vi "test - Arguments or Respsone.vi"(8 "error in (no error)":errorcluster, 11 "TestCase in":refnum<class "testcase-Supported-Datatype.lvclass">) -> (0 "error out":errorcluster, 3 "TestCase out":refnum<class "testcase-Supported-Datatype.lvclass">)   [LabVIEW 2017, in "testcase-Supported-Datatype.lvclass"]
uses:
  testcase-Supported-Datatype.lvclass
  3126c190-a873-4347-b4f7-a4a9805c9280.vi
  c9e66315-a3dc-45cf-9eb3-a329de137435.vi
  5e45644a-04d9-431d-85da-59447771591c.vi
  acccb231-0f0e-4c8a-8d12-71726bcd94d5.vi
  addons/API-String-Arugments-Support/_Support/Convert API String Arguments to Data(variant).vi
  <vilib>/addons/_JKI Toolkits/VI Tester/TestCase.llb/TestCase.lvclass
  C:/Program Files (x86)/National Instruments/LabVIEW 2017/vi.lib/addons/_JKI Toolkits/VI Tester/TestCase.llb/TestCase.lvclass
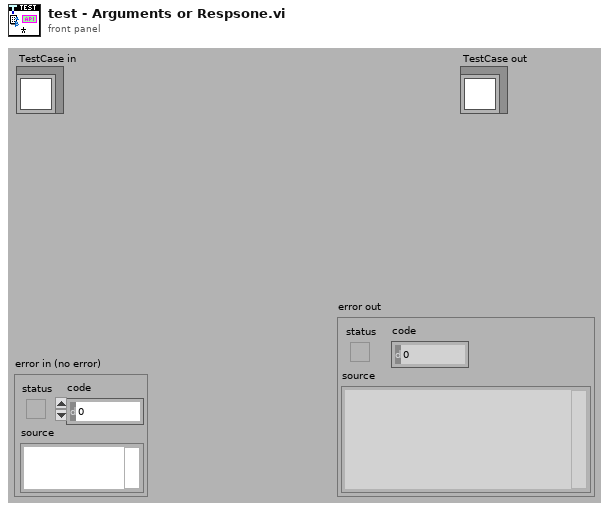
[diagram p1: front panel]
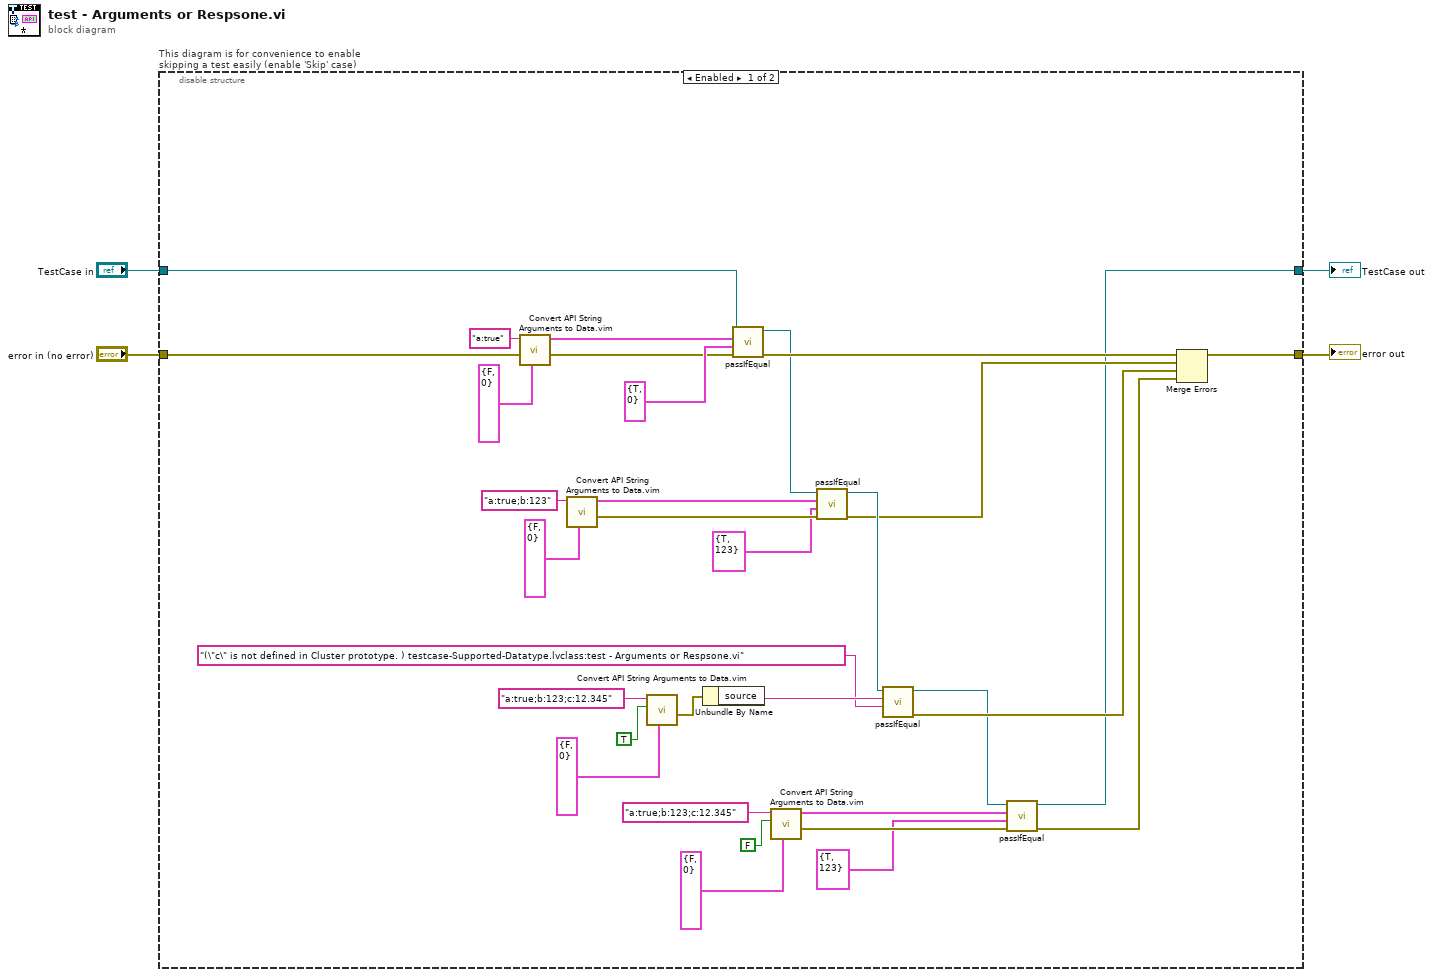
[diagram p0: block diagram]
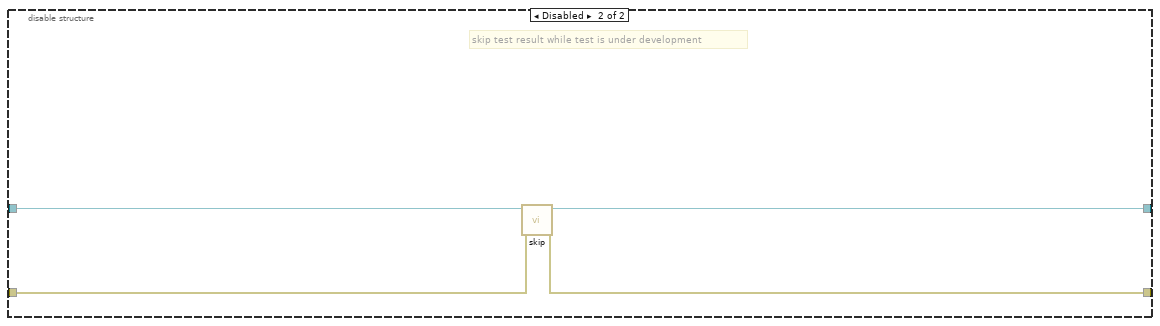
[diagram p2: hidden frame]
diagram:
  n1 = disable-structure "This diagram is for convenience to enable skipping a test easily (enable 'Skip' case)" shown="Enabled" {
    disable-tunnel: "TestCase in" -> [w37 w41]
    disable-tunnel: [w9 w39] -> w1
    disable-tunnel: [w36 w40] -> w3
    disable-tunnel: "error in (no error)" -> [w25 w38]
    frame Enabled {
      n2 = call "Convert API String Arguments to Data.vim"("Reference Type"=cluster{"a":bool, "b":i32} {"a"=FALSE, "b"=0}, "error in (no error)"=w25, "API String"="a:true" ("String")) -> ("error out"=w27:errorcluster, "Data"=w29:cluster{"a":bool, "b":i32})  [unwired: 5 in]
      n3 = call "Convert API String Arguments to Data.vim"("Reference Type"=cluster{"a":bool, "b":i32} {"a"=FALSE, "b"=0}, "API String"="a:true;b:123" ("String")) -> ("error out"=w22:errorcluster, "Data"=w20:cluster{"a":bool, "b":i32})  [unwired: 6 in]
      n4 = call "Convert API String Arguments to Data.vim"("Reference Type"=cluster{"a":bool, "b":i32} {"a"=FALSE, "b"=0}, "Strict Label Check? (T)"=TRUE ("Strict Label Check?(T)"), "API String"="a:true;b:123;c:12.345" ("String")) -> ("error out"=w7:errorcluster)  [unwired: 5 in, 1 out]
      n5 = Unbundle By Name(w7) -> ("source"=w6:string)
      n6 = call-dynamic "passIfEqual.vi"("error in (no error)"=w27, "y"=cluster{"a":bool, "b":i32} {"a"=TRUE, "b"=0} ("Data"), "x"=w29, "TestCase in"=w37) -> ("error out"=w26:errorcluster, "TestCase out"=w24:refnum<class "testcase-Supported-Datatype.lvclass">)  [unwired: 6 in]
      n7 = call "Convert API String Arguments to Data.vim"("Reference Type"=cluster{"a":bool, "b":i32} {"a"=FALSE, "b"=0}, "Strict Label Check? (T)"=FALSE ("Strict Label Check?(T)"), "API String"="a:true;b:123;c:12.345" ("String")) -> ("error out"=w15:errorcluster, "Data"=w13:cluster{"a":bool, "b":i32})  [unwired: 5 in]
      n8 = call-dynamic "passIfEqual.vi"("error in (no error)"=w22, "y"=cluster{"a":bool, "b":i32} {"a"=TRUE, "b"=123} ("Data 2"), "x"=w20, "TestCase in"=w24) -> ("error out"=w18:errorcluster, "TestCase out"=w23:refnum<class "testcase-Supported-Datatype.lvclass">)  [unwired: 6 in]
      n9 = call-dynamic "passIfEqual.vi"("y"="(\"c\" is not defined in Cluster prototype. ) testcase-Supported-Datatype.lvclass:test - Arguments or Respsone.vi" ("source"), "x"=w6, "TestCase in"=w23) -> ("error out"=w19:errorcluster, "TestCase out"=w10:refnum<class "testcase-Supported-Datatype.lvclass">)  [unwired: 7 in]
      n10 = call-dynamic "passIfEqual.vi"("error in (no error)"=w15, "y"=cluster{"a":bool, "b":i32} {"a"=TRUE, "b"=123} ("Data 3"), "x"=w13, "TestCase in"=w10) -> ("error out"=w8:errorcluster, "TestCase out"=w9:refnum<class "testcase-Supported-Datatype.lvclass">)  [unwired: 6 in]
      n11 = Merge Errors(w26, w18, w19, w8) -> (w36:errorcluster)
    }
    frame Disabled {
      # "skip test result while test is under development"
      n12 = call <vilib>:"skip.vi"("error in (no error)"=w38, "TestCase in"=w41) -> ("error out"=w40:errorcluster, "TestCase out"=w39:refnum<class "testcase-Supported-Datatype.lvclass">)  [unwired: 8 in]
    }
  }
  "error out" <- w3
  "TestCase out" <- w1
